vi "CAENHV Set Sys Prop Numeric.vi"(8 "error in (no error)":errorcluster, 9 "Set":i16, 10 "PropName":string, 11 "handle":i32) -> (0 "error out":errorcluster)   [LabVIEW 2009, in "CAENHVWrapper.lvlib"]
doc: "CAENHVLIB_API CAENHVRESULT CAENHV_SetSysProp(int handle, \n const char *PropName, void *Set);"
uses:
  <userlib>/CAENHVWrapper/CAENHVWrapper.lvlib
  <userlib>/CAENHVWrapper/CAENHVWrapper.dll
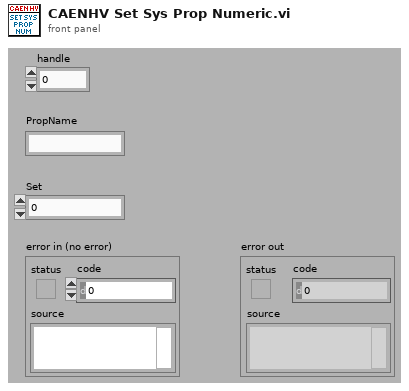
[diagram p1: front panel]
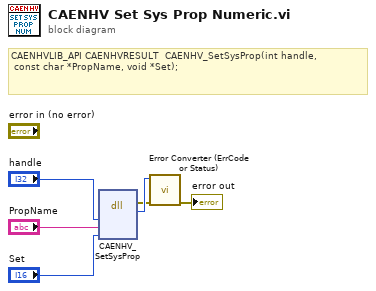
[diagram p0: block diagram]
diagram:
  # "CAENHVLIB_API CAENHVRESULT  CAENHV_SetSysProp(int handle, \n const char\t*PropName, void *Set);"
  n1 = dll-call lib="C:/Program Files/National Instruments/LabVIEW 2009/user.lib/CAENHVWrapper/CAENHVWrapper.*" fn="CAENHV_SetSysProp"("handle"="handle", "PropName"="PropName", "Set"="Set") -> (error out=w5:errorcluster, "return type"=w6:u16)  [unwired: 6 in, 1 out]
  n2 = call <userlib>:"Error Converter (ErrCode or Status).vi"("error in (no error)"=w5, "error code"=w6) -> ("error out"=→"error out":errorcluster)  [unwired: 9 in]
